vi "HandlePass.vi"(8 "error in (no error)":errorcluster, 10 "Perform?":bool, 11 "DoubleClick?":bool) -> (0 "error out":errorcluster, 1 "Call?":bool, 2 "PassState":T2=enum."Pass", 3 "PassType":T1)   [LabVIEW 2015]
doc: "Determines which pass to perform, their state, and whether to actually call the pass VI.\n\nThe ground pass is activated with a single click (<B>DoubleClick?</B> = F), and reset with a single click.\nThe elevated pass is activated with a double click (<B>DoubleClick</B> = T) and reset with a double click."
uses:
  PassState.ctl
  PassType.ctl
  HandlePassAction.ctl
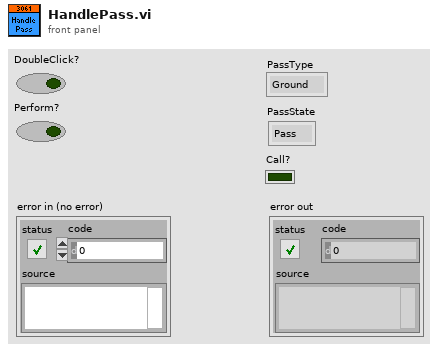
[diagram p1: front panel]
types:
  T1 = typedef "PassType.ctl" = enum16{"Ground", "Elevated"}
  T2 = typedef "PassState.ctl" = enum16{"Stop", "Pass"}
  T3 = typedef "HandlePassAction.ctl" = enum16{"Idle", "Ground", "Elevated"}
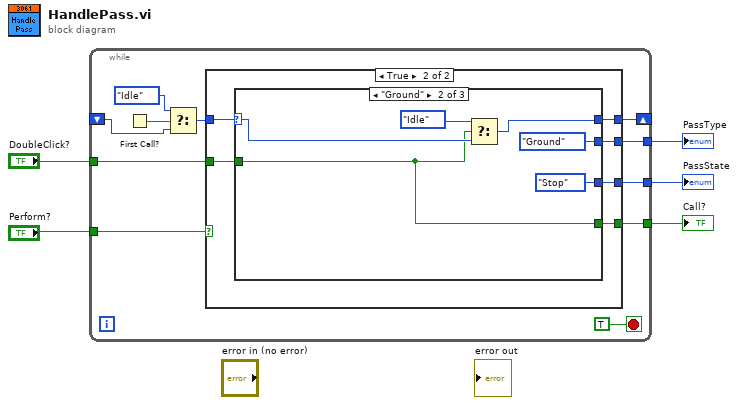
[diagram p0: block diagram]
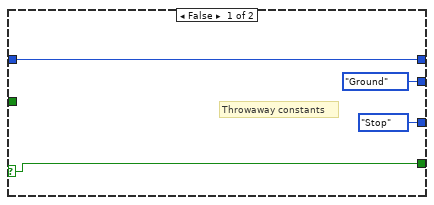
[diagram p2: hidden frame]
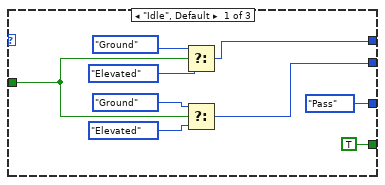
[diagram p3: hidden frame]
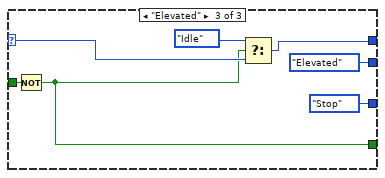
[diagram p4: hidden frame]
diagram:
  n1 = while {
    tunnel: "Perform?" -> [w15]
    shift-right: [w14] -> _
    shift-left: _ -> [w11]
    tunnel: "DoubleClick?" -> [w9]
    tunnel: [w8] -> w3
    tunnel: [w7] -> w2
    tunnel: [w6] -> w1
    stop <- TRUE stop-if-true
    n2 = First Call?() -> (First Call?: T/F=w12:bool)
    n3 = Select(t=HandlePassAction."Idle", s=w12, f=w11) -> (s? t:f=w10:T3)
    n4 = case shown="True" w15 {
      selector: w15 -> [w19 _]
      tunnel: w10 -> [w20 w26]
      tunnel: [w20 w24] -> w14
      tunnel: w9 -> [_ w25]
      tunnel: [PassType."Ground" ("PassType") w23] -> w8
      tunnel: [PassState."Stop" ("PassState") w22] -> w7
      tunnel: [w19 w21] -> w6
      frame False {
        # "Throwaway constants"
      }
      frame True {
        n5 = case shown="\"Ground\"" w26 {
          selector: w26 -> [_ w37 w45]
          tunnel: w25 -> [w29 w36 w44]
          tunnel: [w35 w38 w43] -> w24
          tunnel: [w30 PassType."Ground" ("PassType") PassType."Elevated" ("PassType")] -> w23
          tunnel: [PassState."Pass" ("PassState") PassState."Stop" ("PassState") PassState."Stop" ("PassState")] -> w22
          tunnel: [TRUE w36 w42] -> w21
          frame "Idle", Default {
            n6 = Select(t=HandlePassAction."Ground", s=w29, f=HandlePassAction."Elevated") -> (s? t:f=w35:T3)
            n7 = Select(t=PassType."Ground" ("PassType"), s=w29, f=PassType."Elevated" ("PassType")) -> (s? t:f=w30:T1)
          }
          frame "Ground" {
            n8 = Select(t=HandlePassAction."Idle", s=w36, f=w37) -> (s? t:f=w38:T3)
          }
          frame "Elevated" {
            n9 = Not(x=w44) -> (.not. x?=w42:bool)
            n10 = Select(t=HandlePassAction."Idle", s=w42, f=w45) -> (s? t:f=w43:T3)
          }
        }
      }
    }
  }
  "PassState" <- w2
  "PassType" <- w3
  "Call?" <- w1
